vi "Destroy.vi"(8 "error in (no error)":errorcluster, 11 "Int16Array in":refnum<class "Int16Array.lvclass">) -> (0 "error out":errorcluster)   [LabVIEW 2012, in "MDSplus.lvlib" / "Int16Array.lvclass"]
uses:
  <vilib>/MDSplus/Classes/Data_Class/Array_Class/Int16Array_Class/Int16Array.lvclass
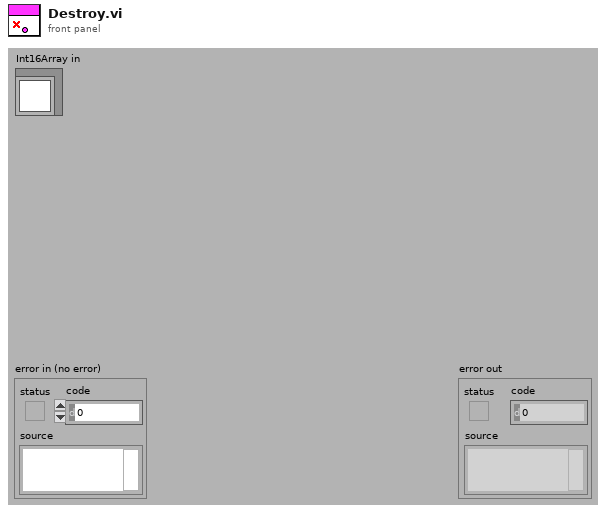
[diagram p1: front panel]
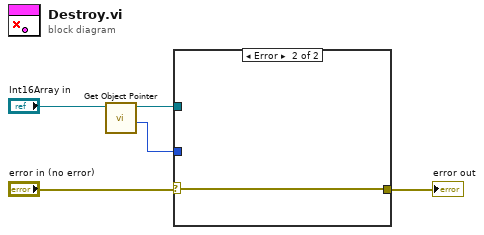
[diagram p0: block diagram]
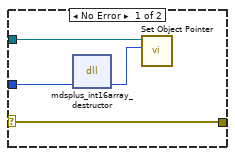
[diagram p2: hidden frame]
diagram:
  n1 = call-dynamic "Get Object Pointer.vi"("Data in"="Int16Array in") -> ("Object Pointer"=w4:i64, "Data out"=w5:refnum<class "Int16Array.lvclass">)  [unwired: 8 in, 1 out]
  n2 = case shown="Error" "error in (no error)" {
    selector: "error in (no error)" -> [w6 w10]
    tunnel: w5 -> [w9 _]
    tunnel: w4 -> [w8 _]
    tunnel: [w6 w10] -> w2
    frame No Error {
      n3 = dll-call lib="MDSobjectsLVShr" fn="mdsplus_int16array_destructor"("lvInt16ArrayPtr"=w8) -> ("lvInt16ArrayPtr"=w7:i64)  [unwired: 4 in, 2 out]
      n4 = call-dynamic "Set Object Pointer.vi"("Object Pointer"=w7, "Data in"=w9) -> ()  [unwired: 9 in, 1 out]
    }
    frame Error {
    }
  }
  "error out" <- w2
